vi "AUTON_Choose_File.vi"(10 "Joystick 2 Refnum":string, 11 "Joystick 1 Refnum":string) -> (1 "Auton File":dbl, 2 "Refresh":bool, 3 "Allow Change":bool)   [LabVIEW 2012]
uses:
  <vilib>/Rock Robotics/WPI/Joystick/WPI_JoystickGetSetRefNum.vi
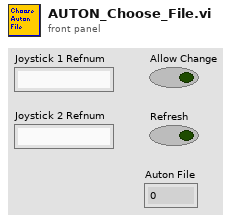
[diagram p1: front panel]
types:
  T1 = typedef "WPI_JoystickDevRef.ctl" = cluster{"Device":T2}
  T2 = typedef "WPI_JoystickDeviceEnum.ctl" = enum16{"USB 1", "USB 2", "USB 3", "USB 4", "Kinect 1", "Kinect 2"}
  T3 = typedef "WPI_JoystickButtonState.ctl" = cluster{"Button 1":bool, "Button 2":bool, "Button 3":bool, "Button 4":bool, "Button 5":bool, "Button 6":bool, "Button 7":bool, "Button 8":bool, "Button 9":bool, "Button 10":bool, "Button 11":bool, "Button 12":bool}
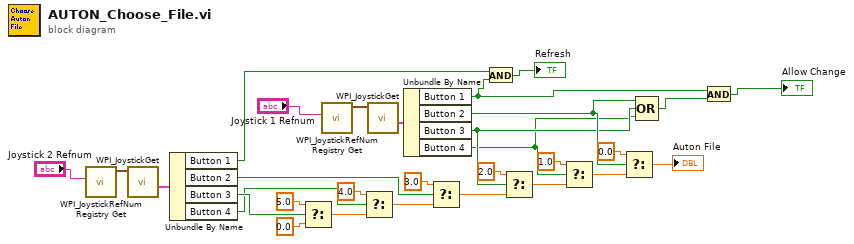
[diagram p0: block diagram]
diagram:
  n1 = call <vilib>:"WPI_JoystickRefNum Registry Get.vi"("refnum name"="Joystick 2 Refnum") -> ("JoystickDevRef"=w11:T1)  [unwired: 9 in, 1 out]
  n2 = call <vilib>:"WPI_JoystickGet.vi"("JoystickDevRef"=w11) -> ("Buttons"=w13:T3)  [unwired: 4 in, 2 out]
  n3 = Unbundle By Name(w13) -> ("Button 1"=w7:bool, "Button 2"=w22:bool, "Button 3"=w28:bool, "Button 4"=w26:bool)
  n4 = Select(t=5.0, s=w28, f=0.0) -> (s? t:f=w27:dbl)
  n5 = call <vilib>:"WPI_JoystickRefNum Registry Get.vi"("refnum name"="Joystick 1 Refnum") -> ("JoystickDevRef"=w8:T1)  [unwired: 9 in, 1 out]
  n6 = Select(t=4.0, s=w26, f=w27) -> (s? t:f=w24:dbl)
  n7 = call <vilib>:"WPI_JoystickGet.vi"("JoystickDevRef"=w8) -> ("Buttons"=w12:T3)  [unwired: 4 in, 2 out]
  n8 = Unbundle By Name(w12) -> ("Button 1"=w5:bool, "Button 2"=w3:bool, "Button 3"=w2:bool, "Button 4"=w1:bool)
  n9 = Select(t=3.0, s=w22, f=w24) -> (s? t:f=w21:dbl)
  n10 = And(x=w7, y=w5) -> (x .and. y?=→"Refresh":bool)
  n11 = Select(t=2.0, s=w2, f=w21) -> (s? t:f=w16:dbl)
  n12 = Select(t=1.0, s=w1, f=w16) -> (s? t:f=w15:dbl)
  n13 = Select(t=0.0, s=w3, f=w15) -> (s? t:f=→"Auton File":dbl)
  n14 = Compound Arithmetic op=OR(w3, w2, w1) -> (w6:bool)
  n15 = And(x=w5, y=w6) -> (x .and. y?=→"Allow Change":bool)
